vi "Configure Edit Mode.vi"(8 "error in (no error)":errorcluster, 9 "Edit Mode (1)":i16=1 min=0 max=1 step=1, 11 "VISA resource name":refnum<visa-resource-name>) -> (0 "error out":errorcluster, 3 "VISA resource name out":refnum<visa-resource-name>)   [LabVIEW 2012, in "Temptronic TP04300.lvlib"]
doc: "This VI allows to enter and clear the edit mode in TP04300 instrument.\n<b>Edit Mode Flag</b> - used to enter and clear the Edit mode in the instrument\n\nDefault Value: 1\nValid Range: 0-1 \n 1 - enter the edit mode\n 0 - clear the edit mode"
uses:
  <instrlib>/Temptronic TP04300/Temptronic TP04300.lvlib
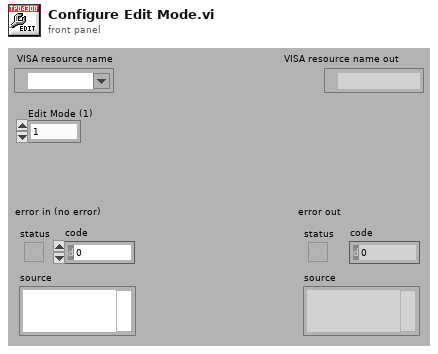
[diagram p1: front panel]
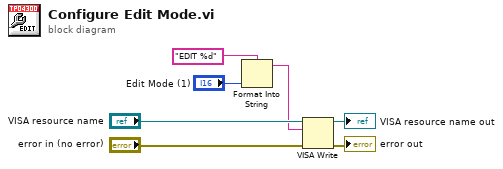
[diagram p0: block diagram]
diagram:
  n1 = Format Into String(format string="EDIT %d", "Edit Mode (1)") -> (resulting string=w3:string)  [unwired: 2 in, 1 out]
  n2 = VISA Write(VISA resource name="VISA resource name", write buffer=w3, error in (no error)="error in (no error)") -> (VISA resource name out=→"VISA resource name out":refnum<visa-resource-name>, error out=→"error out":errorcluster)  [unwired: 1 out]
